vi "BRig_Host__Loop_Producer__tcp_System__Data_storeFiles_v3.vi"(6 "input_n":i32, 8 "input_stored":bool[](array[boolean]), 9 "input_arrPath_target":path[](array[path]), 10 "input_exist_source":bool[](array[boolean]), 11 "input_arrPath_source":path[](array[path])) -> (0 "output_stored":bool[](array[boolean]))   [LabVIEW 2014]
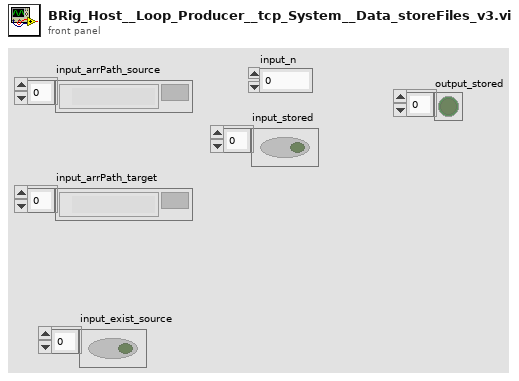
[diagram p1: front panel]
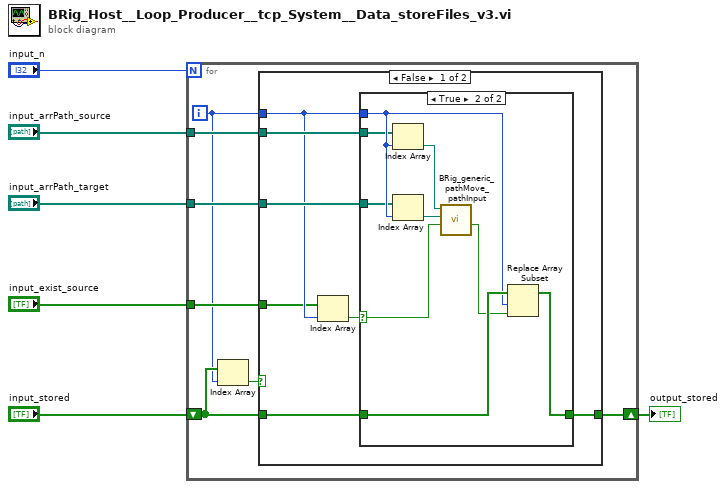
[diagram p0: block diagram]
diagram:
  n1 = for {
    N: "input_n" -> [_]
    tunnel: "input_arrPath_source" -> [w13]
    tunnel: "input_arrPath_target" -> [w12]
    tunnel: "input_exist_source" -> [w10]
    shift-right: [w11] -> w1
    shift-left: "input_stored" -> [w9]
    i -> [w8]
    n2 = Index Array(array=w9, index=w8) -> (element=w7:bool)
    n3 = case shown="False" w7 {
      tunnel: w13 -> [w20 _]
      tunnel: w12 -> [w19 _]
      tunnel: w9 -> [w18 w31]
      tunnel: [w17 w31] -> w11
      tunnel: w8 -> [w16 _]
      tunnel: w10 -> [w15 _]
      frame False {
        n4 = Index Array(array=w15, index=w16) -> (element=w14:bool)
        n5 = case shown="True" w14 {
          selector: w14 -> [_ w28]
          tunnel: w16 -> [_ w25]
          tunnel: w20 -> [_ w23]
          tunnel: w19 -> [_ w24]
          tunnel: w18 -> [w21 w27]
          tunnel: [w21 w26] -> w17
          frame False {
          }
          frame True {
            n6 = Index Array(array=w23, index=w25) -> (element=w29:path)
            n7 = Index Array(array=w24, index=w25) -> (element=w30:path)
            n8 = call "BRig_generic_pathMove_pathInput.vi"("input_Ioverwrite"=w28, "input_filePath_target"=w30, "input_filePath_source"=w29) -> ("output_Iexist"=w22:bool)  [unwired: 6 in, 2 out]
            n9 = Replace Array Subset(array=w27, new element=w22, index=w25) -> (w26:bool[])
          }
        }
      }
      frame True {
      }
    }
  }
  "output_stored" <- w1
